vi "FTW-TransferClient-Destroy.vi"(0 "Transfer Client":refnum<k24>, 11 "error in":errorcluster) -> (15 "error out":errorcluster)   [LabVIEW 2015]
panel:
  # "Inputs"
  # "Outputs"
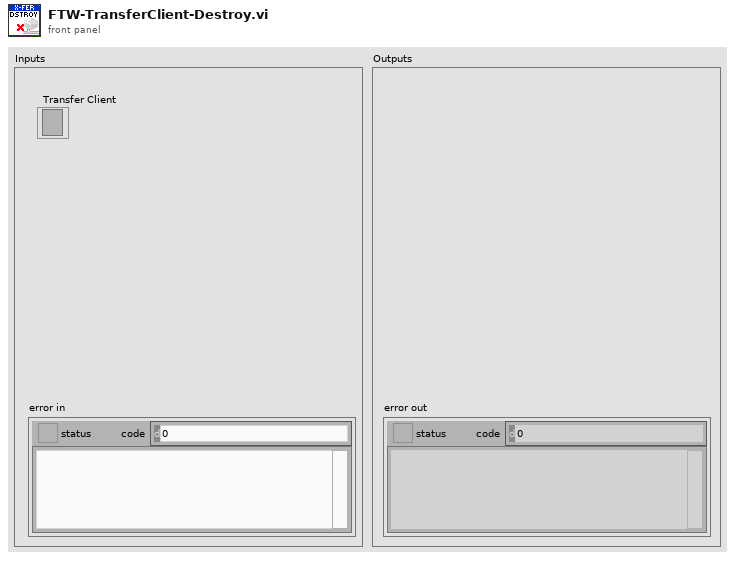
[diagram p1: front panel]
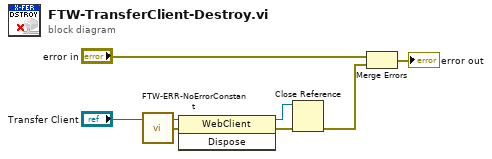
[diagram p0: block diagram]
diagram:
  n1 = call "FTW-ERR-NoErrorConstant.vi"() -> ("no error"=w1:errorcluster)
  n2 = invoke class="WebClient" method="Dispose"(reference="Transfer Client", error in=w1) -> (reference out=w5:refnum<k24>, error out=w4:errorcluster)  [unwired: 1 in, 1 out]
  n3 = Close Reference(reference=w5, error in (no error)=w4) -> (error out=w3:errorcluster)
  n4 = Merge Errors("error in", w3) -> (→"error out":errorcluster)
